vi "Teleop.vi"() -> (1 "Stop program and write to file":bool=TRUE, 2 "SWITCH TO AUTONOMOUS":bool=TRUE, 3 "output cluster":T1)   [LabVIEW 2014]
panel:
  in  "Pyramid":string(combo)="No Attempt"
  in  "Where do they pick up discs?":string(combo)="None"
  in  "Stop Program and Write to File":bool
  in  "SWITCH TO AUTONOMOUS":bool=TRUE
  in  "Comments":string
  in  "Missed Shots":dbl
  in  "5 Points":dbl
  in  "1 Point":dbl
  in  "3 Points":dbl
  in  "2 Points":dbl
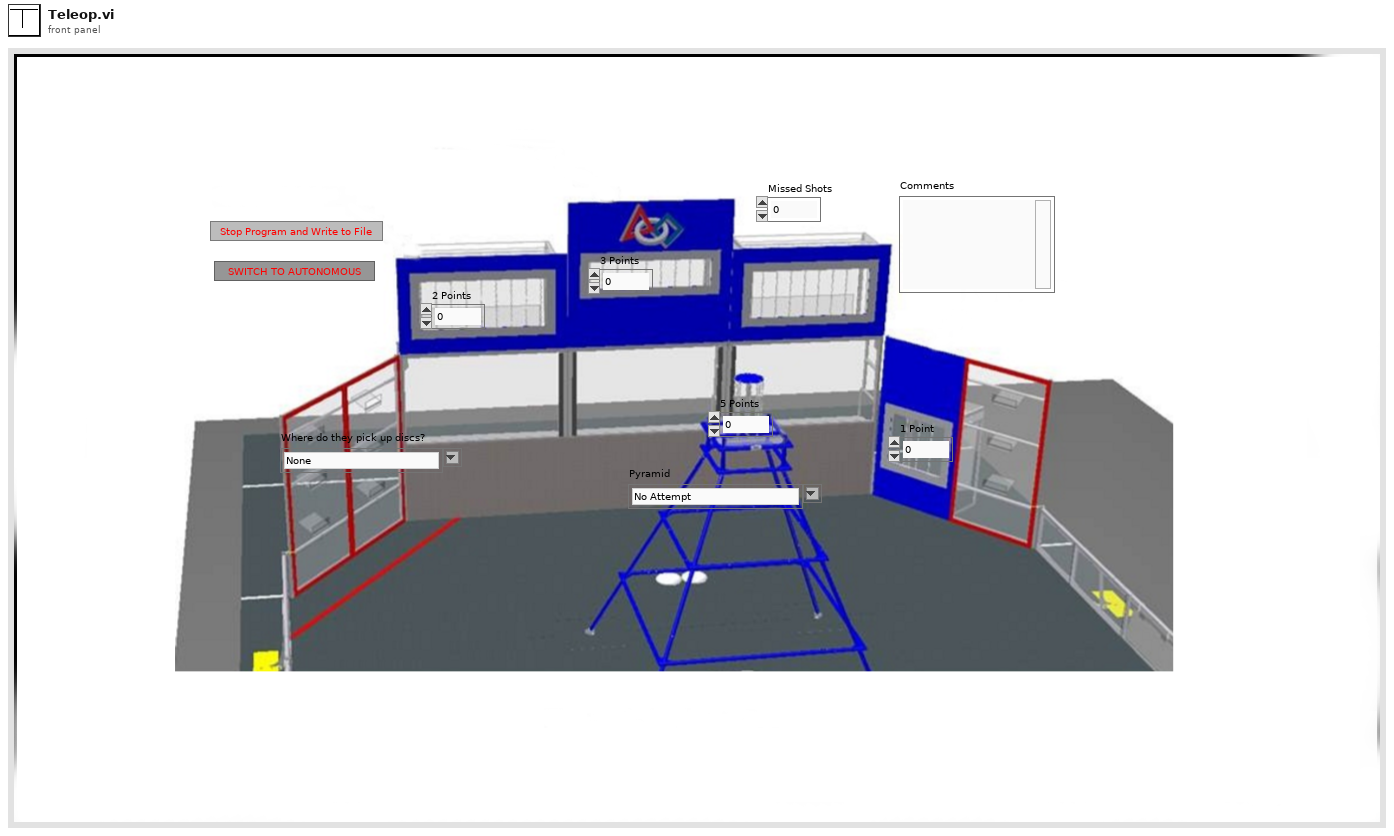
[diagram p1: front panel]
types:
  T1 = cluster{"1 Point":dbl, "2 Points":dbl, "3 Points":dbl, "5 Points":dbl, "Where do they pick up discs?":string, "Comments":string, "Missed Shots":dbl, "Pyramid":string, "Total":dbl}
  T2 = cluster{"1 Point":dbl, "2 Points":dbl, "3 Points":dbl, "5 Points":dbl, "Where do they pick up discs?":string, "Comments":string, "Missed Shots":dbl, "Pyramid":string, dbl}
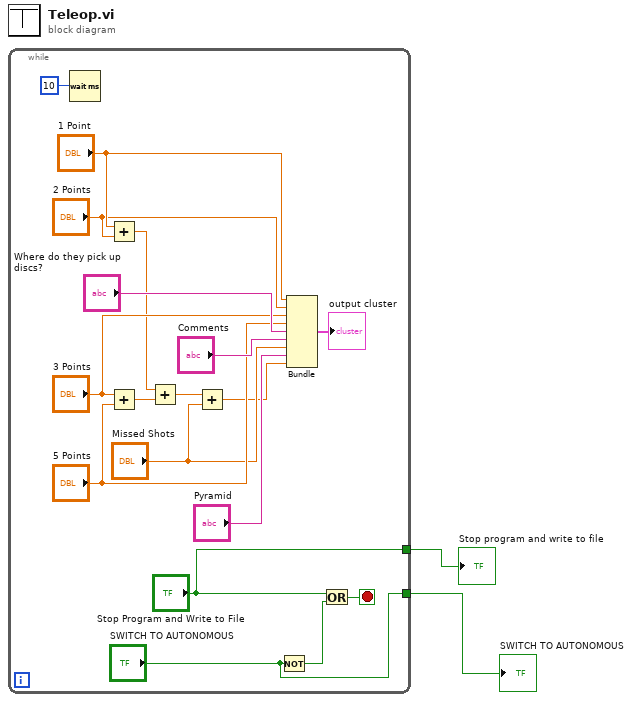
[diagram p0: block diagram]
diagram:
  n1 = while {
    tunnel: ["Stop Program and Write to File"] -> w2
    tunnel: ["SWITCH TO AUTONOMOUS"] -> w1
    stop <- w18 stop-if-true
    n2 = Wait (ms)(milliseconds to wait=u32 10) -> ()  [unwired: 1 out]
    n3 = Add(x="1 Point", y="2 Points") -> (x+y=w8:dbl)
    n4 = Add(x="3 Points", y="5 Points") -> (x+y=w7:dbl)
    n5 = Add(x=w8, y=w7) -> (x+y=w5:dbl)
    n6 = Add(x=w5, y="Missed Shots") -> (x+y=w4:dbl)
    n7 = Not(x="SWITCH TO AUTONOMOUS") -> (.not. x?=w16:bool)
    n8 = Bundle("1 Point"="1 Point", "2 Points"="2 Points", "3 Points"="3 Points", "5 Points"="5 Points", "Where do they pick up discs?"="Where do they pick up discs?", "Comments"="Comments", "Missed Shots"="Missed Shots", "Pyramid"="Pyramid", w4) -> (→"output cluster":T2)  [unwired: 1 in]
    n9 = Or(x="Stop Program and Write to File", y=w16) -> (x .or. y?=w18:bool)
  }
  "Stop program and write to file" <- w2
  "SWITCH TO AUTONOMOUS" <- w1
